vi "Parse 8.vi"(11 "stream in":u8[](array[numeric])) -> (0 "value":u8, 3 "stream out":u8[](array[numeric]))   [LabVIEW 2015]
doc: "Read an unsigned 8-bit value from a UART data stream."
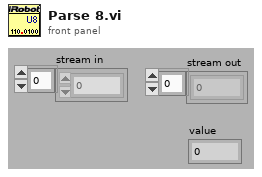
[diagram p1: front panel]
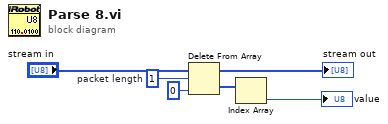
[diagram p0: block diagram]
diagram:
  w4 = 1  # packet length
  n1 = Delete From Array(array="stream in", length=w4, index=0) -> (deleted portion=w3:u8[], array with subset deleted=→"stream out":u8[])
  n2 = Index Array(array=w3) -> (element=→"value":u8)  [unwired: 1 in]
